vi "From Sentence DualHeading(SubVI).vi"(11 "Extract Sentence":string) -> (2 "Parse Data Array":string[](array[string]), 3 "Time Data Array":string[](array[string]))   [LabVIEW 2019]
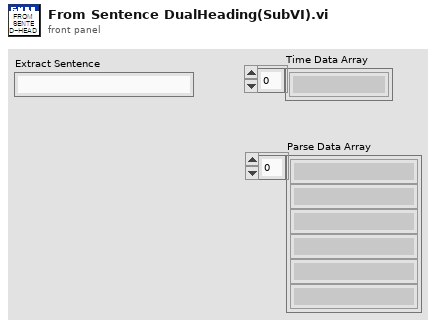
[diagram p1: front panel]
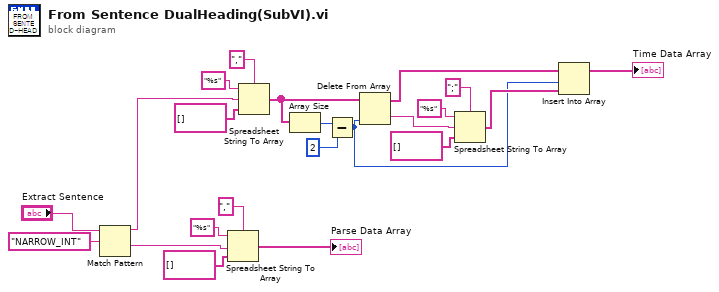
[diagram p0: block diagram]
diagram:
  n1 = Match Pattern(string="Extract Sentence", regular expression="NARROW_INT") -> (before substring=w14:string, after substring=w18:string)  [unwired: 1 in, 2 out]
  n2 = Spreadsheet String To Array(delimiter (Tab)="," ("regular expression"), format string="%s", spreadsheet string=w18, array type (2D Dbl)=string[] []) -> (array=→"Parse Data Array":string[])
  n3 = Spreadsheet String To Array(delimiter (Tab)="," ("regular expression"), format string="%s", spreadsheet string=w14, array type (2D Dbl)=string[] []) -> (array=w12:string[])
  n4 = Array Size(array=w12) -> (size(s)=w4:i32)
  n5 = Subtract(x=w4, y=2) -> (x-y=w2:i32)
  n6 = Delete From Array(array=w12, index=w2) -> (deleted portion=w8:string, array with subset deleted=w7:string[])  [unwired: 1 in]
  n7 = Spreadsheet String To Array(delimiter (Tab)=";" ("regular expression"), format string="%s", spreadsheet string=w8, array type (2D Dbl)=string[] []) -> (array=w6:string[])
  n8 = Insert Into Array(array=w7, index=w2, new element=w6) -> (→"Time Data Array":string[])
